vi "DetermineRegimeDynamicTest.vi"() -> ()   [LabVIEW 2013]
uses:
  Data/TypeDefs/Boat Regimes.ctl
  Data/TypeDefs/Sailing Regimes.ctl
  Data/TypeDefs/Emergency Regimes.ctl
panel:
  out "Heartbeat":bool
  in  "Loop period (ms)":u32(knob) scale=0.0..500.0
  out "Last Commanded Boat Regime":T1
  in  "Trusted Absolute Wind Data (deg) 2":dbl(knob)
  in  "Robot Heading (deg)":dbl(knob)
  out "Commanded Boat Regime":T1
  in  "Desired Heading (deg)":dbl(knob)
  in  "stop":bool
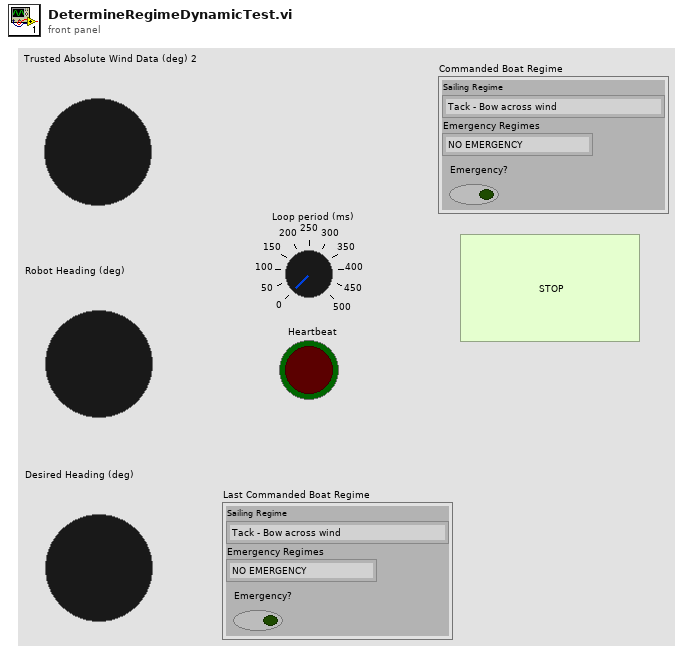
[diagram p1: front panel]
types:
  T1 = typedef "Boat Regimes.ctl" = cluster{"Sailing Regime":T2, "Emergency Regimes":T3, "Emergency?":bool}
  T2 = typedef "Sailing Regimes.ctl" = enum16{"Tack - Bow across wind", "Upwind - Starboard Tack", "Turn between Upwind/Reach - Starboard Tack", "Reach - Starboard Tack", "Turn between Reach/Run - Starboard Tack", "Run - Starboard Tack", "Jibe - Stern across wind", "Run - Port Tack", "Turn between Reach/Run - Port Tack", "Reach - Port Tack", "Turn between Upwind/Reach - Port Tack", "Upwind - Port Tack"}
  T3 = typedef "Emergency Regimes.ctl" = enum16{"NO EMERGENCY", "No Knockdown", "Obstacle Avoid"}
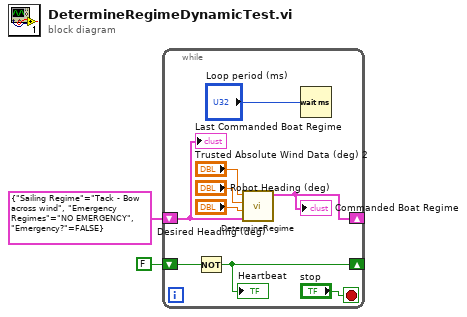
[diagram p0: block diagram]
diagram:
  n1 = while {
    shift-right: [w7] -> _
    shift-left: T1 {"Sailing Regime"=enum."Tack - Bow across wind", "Emergency Regimes"=enum."NO EMERGENCY", "Emergency?"=FALSE} ("Commanded Boat Regime") -> [w6]
    shift-right: [w3] -> _
    shift-left: FALSE -> [w4]
    stop <- "stop" stop-if-true
    n2 = Not(x=w4) -> (.not. x?=w3:bool)
    "Heartbeat" <- w3
    n3 = call "DetermineRegime.vi"("Last Commanded Boat Regime"=w6, "Desired Heading (deg)"="Desired Heading (deg)", "Robot Heading (deg)"="Robot Heading (deg)", "Trusted Absolute Wind Data (deg)"="Trusted Absolute Wind Data (deg) 2") -> ("Commanded Boat Regime"=w7:T1)  [unwired: 7 in]
    "Commanded Boat Regime" <- w7
    n4 = Wait (ms)(milliseconds to wait="Loop period (ms)") -> ()  [unwired: 1 out]
    "Last Commanded Boat Regime" <- w6
  }
